vi "Do.vi"(8 "error in (no error)":errorcluster, 10 "Actor in":refnum<class "Actor.lvclass">, 11 "Actor Data Msg":refnum<class "Observe Data Msg.lvclass">) -> (0 "error out":errorcluster, 2 "Actor out":refnum<class "Actor.lvclass">)   [LabVIEW 2015, in "IObserver.lvlib" / "Observe Data Msg.lvclass"]
doc: "(<B>Filename</B>: Actor Framework.lvlib:Message.lvclass:Do.vi)\n\nDefines what a message does when it is received by an actor. Generally, a message instructs an actor to invoke one of its methods. By default, this method does nothing. A child class must override it to define behavior. Create a child class by using the Actor Framework Message Maker dialog box."
uses:
  Observe Data Msg.lvclass
  <vilib>/ActorFramework/Actor/Actor.lvclass
  IObserver/IObserver.lvclass
  Observe Data Msg.lvclass/Observe Data Msg.ctl
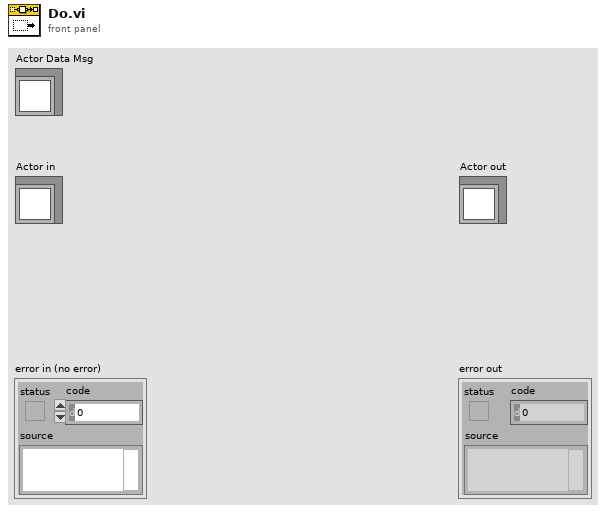
[diagram p1: front panel]
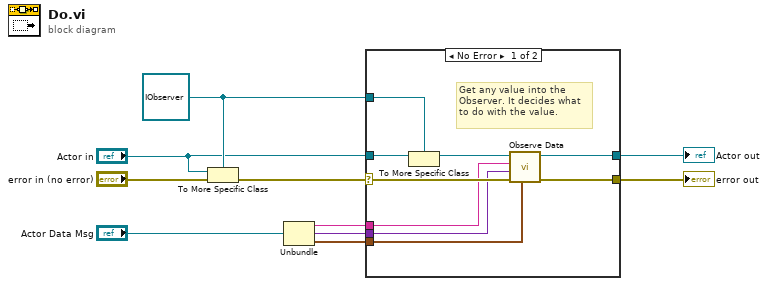
[diagram p0: block diagram]
diagram:
  w9 = refnum<class "IObserver.lvclass"> refnum ("Actor in")
  n1 = To More Specific Class(target class=w9, reference="Actor in", error in="error in (no error)") -> (error out=w10:errorcluster)  [unwired: 1 out]
  n2 = Unbundle("Actor Data Msg") -> (w8:string, w2:variant, w1:timestamp)
  n3 = case shown="No Error" w10 {
    selector: w10 -> [w15 w21]
    tunnel: [w14 w21] -> w6
    tunnel: [w16 w20] -> w4
    tunnel: "Actor in" -> [w19 w20]
    tunnel: w9 -> [w18 _]
    tunnel: w8 -> [w13 _]
    tunnel: w2 -> [w12 _]
    tunnel: w1 -> [w11 _]
    frame No Error {
      # "Get any value into the\nObserver. It decides what\nto do with the value."
      n4 = To More Specific Class(target class=w18, reference=w19) -> (specific class reference=w17:refnum<class "IObserver.lvclass">)  [unwired: 1 in, 1 out]
      n5 = call-dynamic "Observe Data.vi"("Time Stamp"=w11, "error in (no error)"=w15, "Value"=w12, "Datum Name"=w13, "IObserver in"=w17) -> ("error out"=w14:errorcluster, "IObserver out"=w16:refnum<class "IObserver.lvclass">)  [unwired: 5 in]
    }
    frame Error {
      # "If type check fails, pass the\noriginal object out again."
    }
  }
  "error out" <- w6
  "Actor out" <- w4
